vi "Turn Testing.vi"(4 "end angle":u16(ring) items=["0", "45", "90", "135", "180", "225", "270", "315"], 5 "start angle":u16(ring) items=["0", "45", "90", "135", "180", "225", "270", "315"]) -> (3 "x-y":i16)   [LabVIEW 2014]
uses:
  <vilib>/userdefined/High Color/nirio_resource_hc.ctl
  <vilib>/FPGAPlugInAG/myRIO-1900/niLvFpga_Open_myRIO-1900.vi
  <vilib>/rvi/interface/common/dynamic/niFpgaDynamicAddResources.vi
  <vilib>/Utility/error.llb/Error Cluster From Error Code.vi
  <vilib>/rvi/errors/niLvFpgaAdjustHostInterfaceError.vi
  <vilib>/FPGAPlugInAG/Dynamic/niLvFpga_Close_Dynamic.vi
  <vilib>/rvi/interface/nirviOpenFPGA/nirviOpenFPGA.xnode
  FPGA Bitfiles/MITe2015_FPGATarget_FPGA-1900MotorAu_fQqeE40Xepw.lvbitx
  FPGA/FPGA-1900 Motor Automation Test.vi
  <vilib>/rvi/interface/nirviReadWriteControl/nirviReadWriteControl.xnode
  <vilib>/rvi/interface/nirviCloseFPGA/nirviCloseFPGA.xnode
  NiFpgaLv.dll
  <vilib>/rvi/interface/Simulation/niFpgaSimulationCallBeginRW.vi
panel:
  in  "resource name":T1="RIO0"
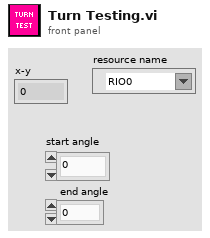
[diagram p1: front panel]
types:
  T1 = typedef "nirio_resource_hc.ctl" = tag
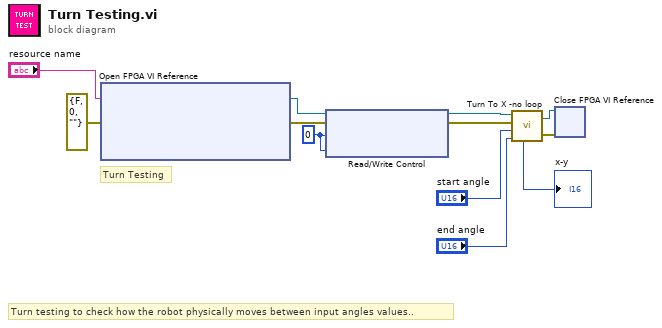
[diagram p0: block diagram]
diagram:
  w9 = i16 0 ("Left Count Length")
  # "Turn testing to check how the robot physically moves between input angles values.."
  # "Turn Testing"
  n1 = xnode "Open FPGA VI Reference"("error in"=errorcluster {"status"=FALSE, "code"=0, "source"=""} ("error out"), "resource name"="resource name") -> ("FPGA VI Reference Out"=w10:refnum<k20>, "error out"=w8:errorcluster)
  n2 = xnode "Read/Write Control"("FPGA VI Reference In"=w10, "error in"=w8, "Left Count Length"=w9, "Right Count Length"=w9) -> ("FPGA VI Reference Out"=w4:refnum<k20>, "error out"=w5:errorcluster)
  n3 = call "Turn To X -no loop.vi"("end angle"="end angle", "start angle"="start angle", "error in"=w5, "FPGA VI Reference in"=w4) -> ("error out"=w2:errorcluster, "FPGA VI Reference Out"=w3:refnum<k20>, "x-y"=→"x-y":i16)  [unwired: 1 in]
  n4 = xnode "Close FPGA VI Reference"("FPGA VI Reference In"=w3, "error in"=w2) -> ()  [unwired: 1 out]
